vi "axc license days to expire.vi"(8 "error in (no error)":errorcluster caption="错误输入（无错误）") -> (0 "error out":errorcluster caption="错误输出", 3 "function return":i32)   [LabVIEW 2015, in "asf_lic.lvlib"]
doc: "AX_LIC_EXPORTS int axc_license_days_to_expire();"
uses:
  asf_lic.lvlib
  asf_lic.dll
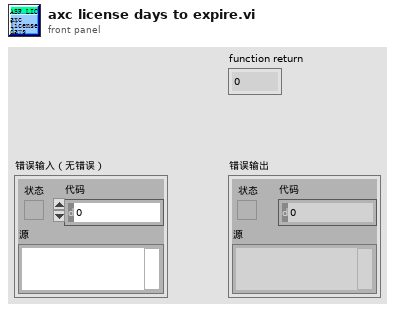
[diagram p1: front panel]
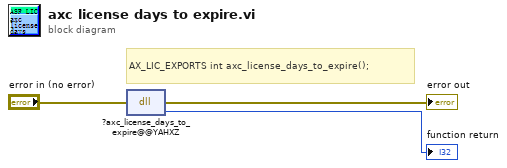
[diagram p0: block diagram]
diagram:
  # "AX_LIC_EXPORTS int axc_license_days_to_expire();"
  n1 = dll-call lib="PTH2>abs CUsersSpesTechDesktopdist-lic函数\tasf_lic.*" fn="?axc_license_days_to_expire@@YAHXZ"(error in="error in (no error)") -> (error out=→"error out":errorcluster, →"function return":i32)  [unwired: 2 in, 1 out]
